vi "Run time (SILAR).vi"(2 "Все время":dbl) -> (0 "Процесс выполнения":dbl(slide) scale=0.0..1.0, 1 "Время выполнения":timestamp format="%<%H:%M:%S>T")   [LabVIEW 2012]
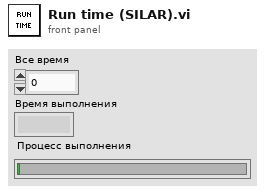
[diagram p1: front panel]
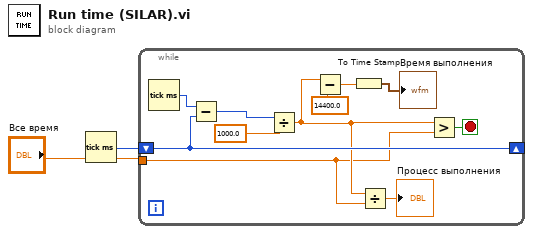
[diagram p0: block diagram]
diagram:
  n1 = Tick Count (ms)() -> (millisecond timer value=w2:u32)
  n2 = while {
    shift-right: [w9] -> _
    shift-left: w2 -> [w9]
    tunnel: "Все время" -> [w4]
    stop <- w10 stop-if-true
    n3 = Tick Count (ms)() -> (millisecond timer value=w13:u32)
    n4 = Subtract(x=w13, y=w9) -> (x-y=w11:u32)
    n5 = Divide(x=w11, y=1000.0) -> (x/y=w5:dbl)
    n6 = Subtract(x=w5, y=14400.0) -> (x-y=w8:dbl)
    n7 = To Time Stamp(1:w8) -> (0:→"Время выполнения":timestamp)
    n8 = Divide(x=w5, y=w4) -> (x/y=→"Процесс выполнения":dbl)
    n9 = Greater?(x=w5, y=w4) -> (0:w10:bool)
  }
